vi "Write Roles.vi"(8 "error in (no error)":errorcluster, 10 "Roles":T1, 11 "StopOffensivePlay in":refnum<class "StopOffensivePlay.lvclass">) -> (0 "error out":errorcluster, 3 "StopOffensivePlay out":refnum<class "StopOffensivePlay.lvclass">)   [LabVIEW 2020, in "StopOffensivePlay.lvclass"]
uses:
  StopOffensivePlay.lvclass
  MarkerRole_class/MarkerRole.lvclass
  AttackerStopRole_class/AttackerStopRole.lvclass
  StopOffensivePlay.lvclass/StopOffensivePlay.ctl
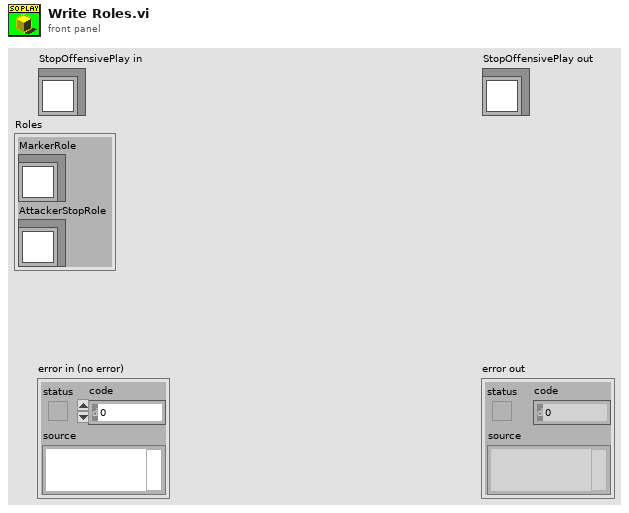
[diagram p1: front panel]
types:
  T1 = cluster{"MarkerRole":refnum<class "MarkerRole.lvclass">, "AttackerStopRole":refnum<class "AttackerStopRole.lvclass">}
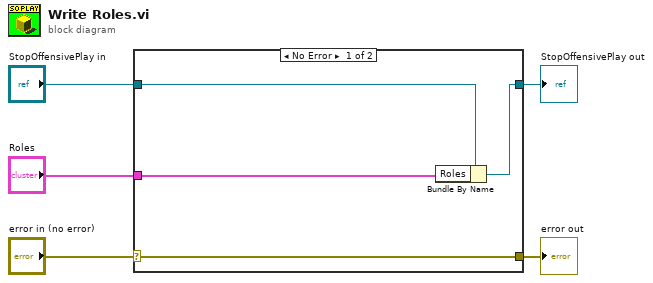
[diagram p0: block diagram]
diagram:
  n1 = case shown="No Error" "error in (no error)" {
    selector: "error in (no error)" -> [w9 w10]
    tunnel: [w9 w10] -> w4
    tunnel: [w7 w11] -> w2
    tunnel: "StopOffensivePlay in" -> [w8 w11]
    tunnel: "Roles" -> [w6 _]
    frame No Error {
      n2 = Bundle By Name(cluster=w8, "Roles"=w6) -> (w7:refnum<class "StopOffensivePlay.lvclass">)
    }
    frame Error {
    }
  }
  "error out" <- w4
  "StopOffensivePlay out" <- w2
